vi "test Event Test Template.vi"(8 "error in (no error)":errorcluster, 11 "TestCase in":refnum<class "VITAC Example Test Case.lvclass">) -> (0 "error out":errorcluster, 3 "TestCase out":refnum<class "VITAC Example Test Case.lvclass">)   [LabVIEW 2015, in "VITAC Example Test Case.lvclass"]
uses:
  VITAC Example Test Case.lvclass
  <vilib>/addons/_JKI Toolkits/VI Tester/TestCase.llb/TestCase.lvclass
panel:
  in  "Numeric":dbl
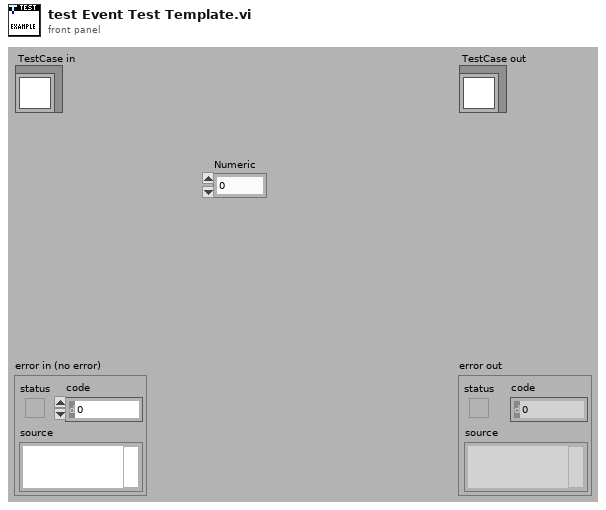
[diagram p1: front panel]
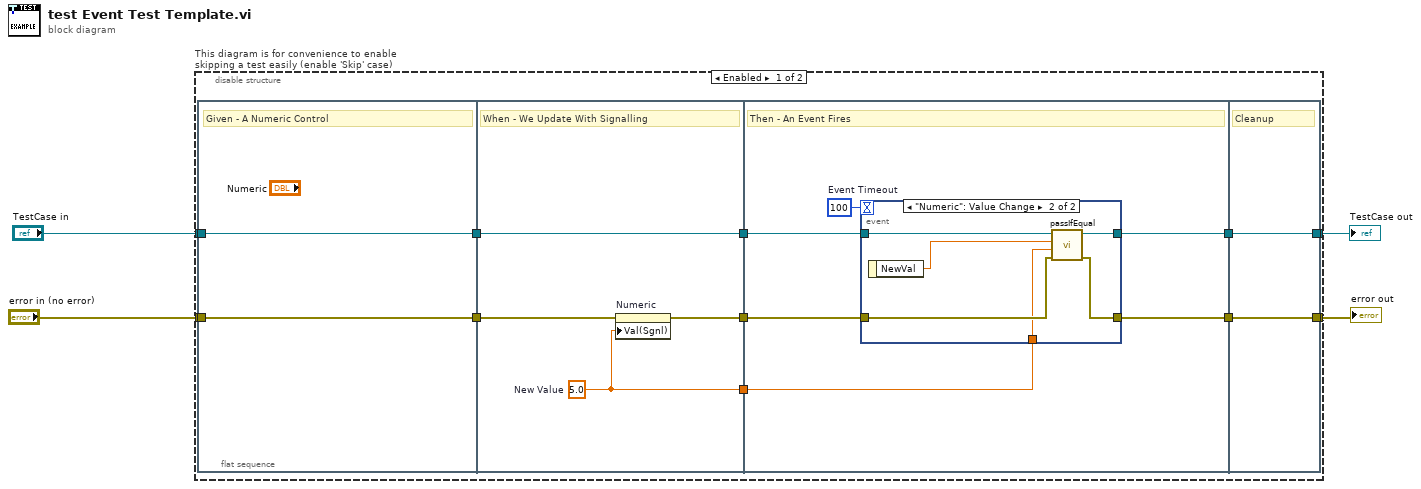
[diagram p0: block diagram]
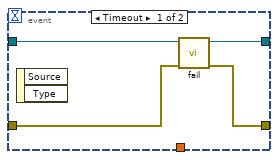
[diagram p2: hidden frame]
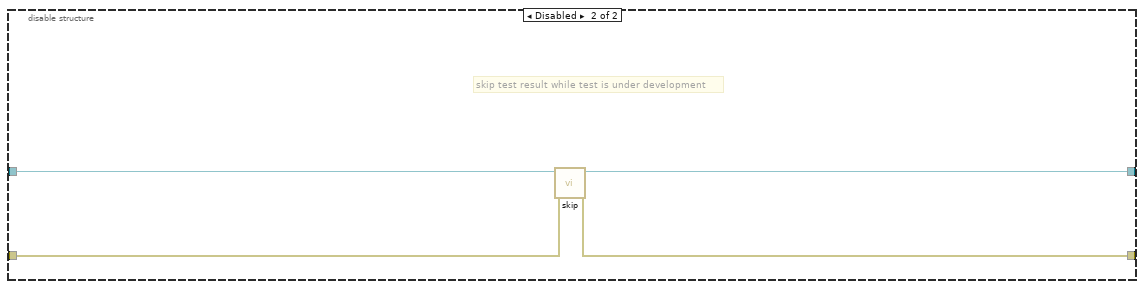
[diagram p3: hidden frame]
diagram:
  n1 = disable-structure "This diagram is for convenience to enable skipping a test easily (enable 'Skip' case)" shown="Enabled" {
    disable-tunnel: "TestCase in" -> [w9 w43]
    disable-tunnel: [w7 w41] -> w1
    disable-tunnel: [w6 w42] -> w3
    disable-tunnel: "error in (no error)" -> [w8 w40]
    frame Enabled {
      n2 = flat-sequence {
        tunnel: w8 -> [w16]
        tunnel: w9 -> [w17]
        tunnel: [w17] -> w15
        tunnel: [w16] -> w14
        tunnel: [w21] -> w13
        tunnel: [w19] -> w12
        tunnel: w15 -> [w21]
        tunnel: w14 -> [w20]
        tunnel: [w18] -> w5
        tunnel: [w26] -> w11
        tunnel: [w23] -> w10
        tunnel: w13 -> [w25]
        tunnel: w12 -> [w24]
        tunnel: w5 -> [w22]
        tunnel: [w38] -> w6
        tunnel: [w39] -> w7
        tunnel: w11 -> [w39]
        tunnel: w10 -> [w38]
        frame #0 {
          # "Given - A Numeric Control"
        }
        frame #1 {
          w18 = 5.0  # New Value
          # "When - We Update With Signalling"
          n3 = property on="Numeric" class="DigNum (strict)"(error in=w20, "Val(Sgnl)"=w18) -> (error out=w19:errorcluster)  [unwired: 1 in, 1 out]
        }
        frame #2 {
          w27 = 100  # Event Timeout
          # "Then - An Event Fires"
          n4 = event shown="[1] \"Numeric\": Value Change" {
            selector: _ -> [_ _]
            dyn-events: _ -> [_ _]
            timeout: w27 -> [_ _]
            tunnel: w25 -> [w31 w37]
            tunnel: [w30 w36] -> w26
            tunnel: [w28 w35] -> w23
            tunnel: w24 -> [w29 w34]
            tunnel: w22 -> [_ w32]
            event Timeout {
              n5 = event-data() -> ()  [unwired: 1 in, 2 out]
              n6 = call-dynamic "fail.vi"("error in (no error)"=w29, "TestCase in"=w31) -> ("error out"=w28:errorcluster, "TestCase out"=w30:refnum<class "VITAC Example Test Case.lvclass">)  [unwired: 8 in]
            }
            event "Numeric": Value Change {
              n7 = event-data() -> ("NewVal"=w33:dbl)  [unwired: 1 in]
              n8 = call-dynamic "passIfEqual.vi"("error in (no error)"=w34, "y"=w32, "x"=w33, "TestCase in"=w37) -> ("error out"=w35:errorcluster, "TestCase out"=w36:refnum<class "VITAC Example Test Case.lvclass">)  [unwired: 6 in]
            }
          }
        }
        frame #3 {
          # "Cleanup"
        }
      }
    }
    frame Disabled {
      # "skip test result while test is under development"
      n9 = call <vilib>:"skip.vi"("error in (no error)"=w40, "TestCase in"=w43) -> ("error out"=w42:errorcluster, "TestCase out"=w41:refnum<class "VITAC Example Test Case.lvclass">)  [unwired: 8 in]
    }
  }
  "error out" <- w3
  "TestCase out" <- w1
